vi "FindItem.vi"(7 "Item Name":string, 8 "error in (no error)":errorcluster, 10 "StructuredDataContainer":variant, 11 "BlueTOMLSerializer in":refnum<class "BlueTOMLSerializer.lvclass">) -> (0 "error out":errorcluster, 1 "Found?":bool, 2 "StructuredDataItem":variant, 3 "BlueTOMLSerializer out":refnum<class "BlueTOMLSerializer.lvclass">)   [LabVIEW 2019, in "BlueTOMLSerializer.lvlib" / "BlueTOMLSerializer.lvclass"]
uses:
  BlueTOMLSerializer.lvclass
  StructuredData.ctl
  Support/TOML Value.ctl
  Support/Key-Value Pair.ctl
  Support/Value.ctl
  Support/Value Type.ctl
  BlueTOMLSerializer.lvlib
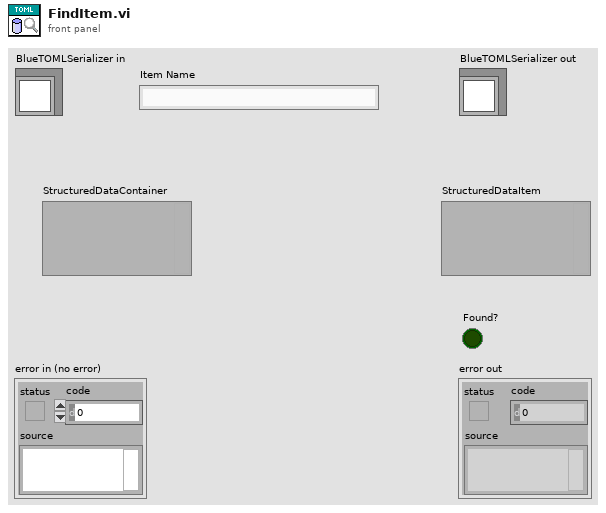
[diagram p1: front panel]
types:
  T1 = typedef "BlueTOMLSerializer.lvlib/BlueTOMLSerializer.lvclass/StructuredData.ctl" = cluster{"TOML Value":T2}
  T2 = typedef "BlueTOMLSerializer.lvlib/TOML Value.ctl" = cluster{"\\type":enum16{"Table", "Array", "String", "Integer", "Float", "Boolean", "Offset Date-Time", "Local Date-Time", "Local Date", "Local Time"}, "ÿýÿýÿýÿýÿýÿþÿýÿýÿý%LV-TOML.lvlib:TOML Key-Value Pair.ctlÿýÿýÿýÿýÿýÿþÿýÿýÿýLV-TOML.lvlib:TOML Value.ctl$":variant}
  T3 = typedef "BlueTOMLSerializer.lvlib/Value.ctl" = cluster{"Type":T4, "Value":variant}
  T4 = typedef "BlueTOMLSerializer.lvlib/Value Type.ctl" = enum16{"Table", "Array", "String", "Integer", "Float", "Boolean", "Offset Date-Time", "Local Date-Time", "Local Date", "Local Time"}
  T5 = typedef "BlueTOMLSerializer.lvlib/Key-Value Pair.ctl" = cluster{"Key":string, "Value":T3}
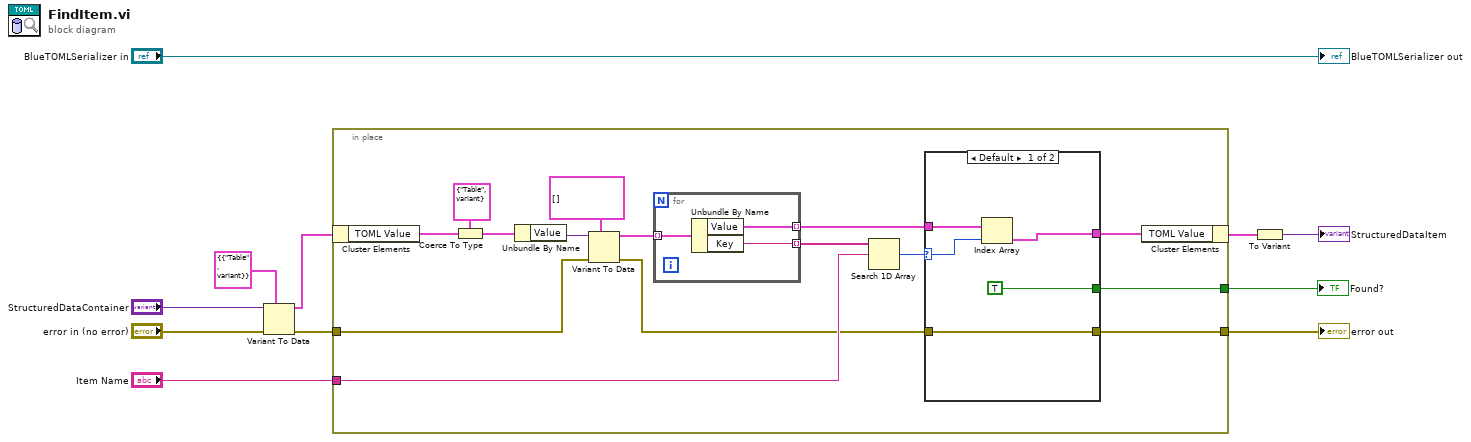
[diagram p0: block diagram]
diagram:
  n1 = Variant To Data(error in="error in (no error)", type=T1 {"TOML Value"={"\\type"=enum."Table", "ÿýÿýÿýÿýÿýÿþÿýÿýÿý%LV-TOML.lvlib:TOML Key-Value Pair.ctlÿýÿýÿýÿýÿýÿþÿýÿýÿýLV-TOML.lvlib:TOML Value.ctl$"=variant}} ("Cluster"), Variant="StructuredDataContainer") -> (data=w9:T1, error out=w3:errorcluster)
  n2 = in-place {
    in-place-border: "Item Name" -> [w19]
    in-place-border: w3 -> [w15]
    in-place-border: [w13] -> w2
    in-place-border: [w12] -> w1
    n3 = in-place-cluster #1(w9) -> ("TOML Value"=w21:T2)
    n4 = Coerce To Type(0:w21, 1:T3 {"Type"=enum."Table", "Value"=variant} ("type")) -> (2:w26:T3)
    n5 = Unbundle By Name(w26) -> ("Value"=w24:variant)
    n6 = Variant To Data(error in=w15, type=T5[] [], Variant=w24) -> (data=w25:T5[], error out=w14:errorcluster)
    n7 = for {
      tunnel: w25 -> [w35] mode=indexing
      tunnel: [w34] -> w17 mode=indexing
      tunnel: [w33] -> w18 mode=indexing
      n8 = Unbundle By Name(w35) -> ("Value"=w34:T3, "Key"=w33:string)
    }
    n9 = Search 1D Array(1D array=w18, element=w19) -> (index of element=w20:i32)  [unwired: 1 in]
    n10 = case shown="Default" w20 {
      selector: w20 -> [w30 _]
      tunnel: w17 -> [w31 _]
      tunnel: [w29 _] -> w16
      tunnel: w14 -> [w28 w32]
      tunnel: [w28 w32] -> w13
      tunnel: [TRUE _] -> w12
      frame Default {
        n11 = Index Array(array=w31, index=w30) -> (element=w29:T3)
      }
      frame -1 {
      }
    }
    n12 = in-place-cluster #1("TOML Value"=w16) -> (w8:T1)
  }
  "error out" <- w2
  "Found?" <- w1
  n13 = To Variant(anything=w8) -> (Variant=→"StructuredDataItem":variant)
  "BlueTOMLSerializer out" <- "BlueTOMLSerializer in"
